vi "Load Device Info.vi"(8 "Error In":errorcluster, 11 "Device Config":T1) -> (0 "Error Out":errorcluster, 3 "Device Config":T1)   [LabVIEW 2014, in "LMH-LINX.lvlib" / "myRIO.lvlib"]
uses:
  <vilib>/MakerHub/LINX/Private/myRIO/myRIO.lvlib
  <vilib>/MakerHub/LINX/Private/Device/Type Defs/LINX Device Config.ctl
  <vilib>/MakerHub/LINX/Private/Type Defs/Interface.ctl
  <vilib>/MakerHub/LINX/Private/Device/Type Defs/TCP Config.ctl
  <vilib>/MakerHub/LINX/Private/Device/Type Defs/Channels.ctl
  <vilib>/MakerHub/LINX/Private/Type Defs/Device Family.ctl
  <vilib>/MakerHub/LINX/LMH-LINX.lvlib
  <vilib>/MakerHub/LINX/Private/Type Defs/Devices - NI.ctl
  <vilib>/MakerHub/LINX/Private/Device/Device.lvlib
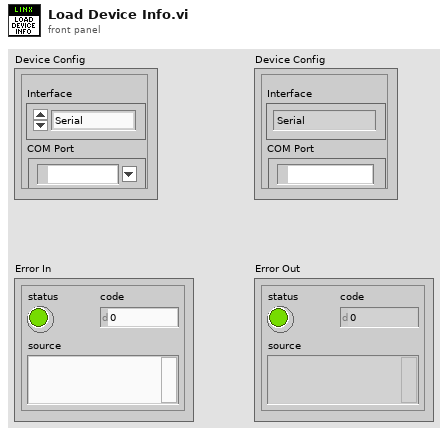
[diagram p1: front panel]
types:
  T1 = typedef "LMH-LINX.lvlib/Device.lvlib/LINX Device Config.ctl" = cluster{"Interface":T2, "COM Port":refnum<visa-resource-name>, "TCP Configuration":T3, "Device Family":u8, "Device ID":u8, "Device Name":string, "TCP Ref":refnum<k5>, "Channels":T4}
  T2 = typedef "LMH-LINX.lvlib/Interface.ctl" = enum16{"Serial", "TCP"}
  T3 = typedef "LMH-LINX.lvlib/Device.lvlib/TCP Config.ctl" = cluster{"IP Address":string, "Port":u16}
  T4 = typedef "LMH-LINX.lvlib/Channels.ctl" = cluster{"DI":u8[], "DO":u8[], "AI":u8[], "AO":u8[], "PWM":u8[], "QE":u8[], "UART":u8[], "I2C 2":u8[], "SPI":u8[], "CAN":u8[], "Servo":u8[], "AI Ref (V)":dbl, "AI Resolution (Bits)":u8, "AO Ref (V)":dbl, "AO Resolution (Bits)":u8}
  T5 = typedef "LMH-LINX.lvlib/Devices - NI.ctl" = enum16{"myRIO-1900", "myRIO-1950"}
  T6 = typedef "LMH-LINX.lvlib/Device Family.ctl" = u8
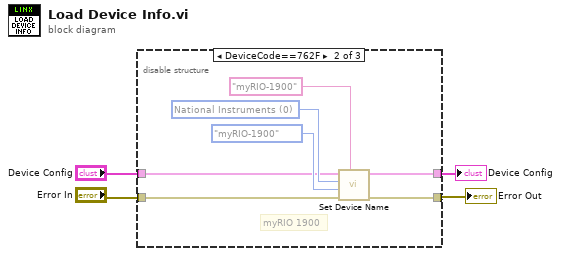
[diagram p0: block diagram]
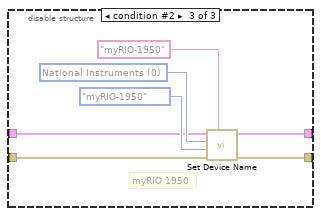
[diagram p3: hidden frame]
diagram:
  n1 = disable-structure shown="DeviceCode==762F" {
    disable-tunnel: [w6 w7 w17] -> w4
    disable-tunnel: "Device Config" -> [w6 w8 w14]
    disable-tunnel: "Error In" -> [w5 w10 w15]
    disable-tunnel: [w5 w9 w16] -> w1
    frame condition #0 (active) {
    }
    frame condition #1 {
      w13 = T6 0 items=["National Instruments", "Digilent", "Arduino"] ("Device Family")
      # "myRIO 1900"
      n2 = call <vilib>:"Set Device Name.vi"("Device Name"="myRIO-1900", "Error In"=w10, "Device ID"=Devices_-_NI."myRIO-1900" ("NI Device"), "Device Family"=w13, "LINX Device Config"=w8) -> ("Error Out"=w9:errorcluster, "LINX Device Config"=w7:T1)  [unwired: 5 in]
    }
    frame condition #2 {
      w18 = T6 0 items=["National Instruments", "Digilent", "Arduino"] ("Device Family")
      # "myRIO 1950"
      n3 = call <vilib>:"Set Device Name.vi"("Device Name"="myRIO-1950", "Error In"=w15, "Device ID"=Devices_-_NI."myRIO-1950" ("NI Device"), "Device Family"=w18, "LINX Device Config"=w14) -> ("Error Out"=w16:errorcluster, "LINX Device Config"=w17:T1)  [unwired: 5 in]
    }
  }
  "Device Config" <- w4
  "Error Out" <- w1
